vi "HandleError.vi"(8 "error in":errorcluster, 10 "origin":string, 11 "Status":i32) -> (0 "error out":errorcluster)   [LabVIEW 2023]
uses:
  <vilib>/Utility/error.llb/whitespace.ctl
  <vilib>/Utility/error.llb/Trim Whitespace One-Sided.vi
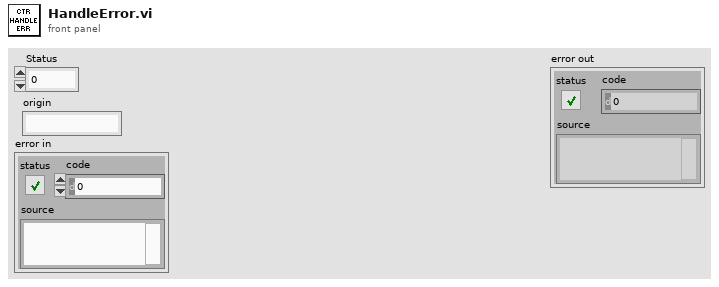
[diagram p1: front panel]
types:
  T1 = typedef "whitespace.ctl" = u16
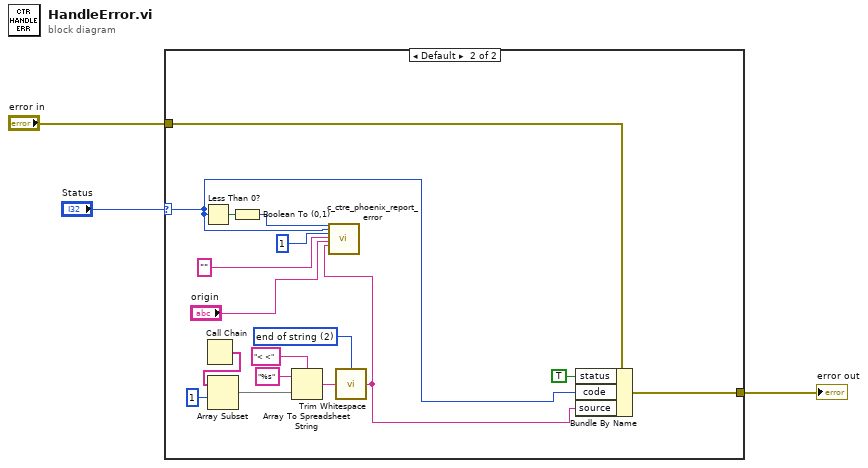
[diagram p0: block diagram]
diagram:
  n1 = case shown="Default" "Status" {
    selector: "Status" -> [_ w8]
    tunnel: "error in" -> [w4 w10]
    tunnel: [w4 w6] -> w1
    frame 0 {
    }
    frame Default {
      w15 = T1 2 items=["both", "start of string", "end of string"] ("location (both)")
      n2 = Less Than 0?(x=w8) -> (x < 0?=w21:bool)
      n3 = Call Chain() -> (call chain=w13:string[])
      n4 = Array Subset(array=w13, index=1) -> (w14:string[])  [unwired: 1 in]
      n5 = Boolean To (0,1)(Boolean=w21) -> (0, 1=w20:i16)
      n6 = Array To Spreadsheet String(delimiter (Tab)="< <", array=w14, 3:"%s" ("format string")) -> (spreadsheet string=w16:string)
      n7 = call <vilib>:"Trim Whitespace.vi"("string"=w16, "location (both)"=w15) -> ("trimmed string"=w7:string)
      n8 = call <vilib>:"c_ctre_phoenix_report_error.vi"("Numeric"=w20, "Numeric 2"=w8, "Numeric 3"=1, "String 2"="", "String 4"="origin", "String 6"=w7) -> ()  [unwired: 19 in, 3 out]
      n9 = Bundle By Name(cluster=w10, "status"=TRUE, "code"=w8, "source"=w7) -> (w6:errorcluster)
    }
  }
  "error out" <- w1
